vi "Action Point_Init.vi"(8 "error in":errorcluster, 11 "Action Point in":refnum<class "Action Point.lvclass">) -> (0 "error out":errorcluster, 3 "Action Point out":refnum<class "Action Point.lvclass">)   [LabVIEW 2024, in "Action Point.lvclass"]
uses:
  Action Point.lvclass
  Config from JSON/Config from JSON.lvclass
  D:/git/HAL/Source/Interfaces/IConfiguration/IConfiguration.lvclass
  Interfaces/IInitialize/IInitialize.lvclass
  Interfaces/ILog Data/ILog Data.lvclass
  Action Point.lvclass/Action Point.ctl
  Interfaces/IConfiguration/IConfiguration.lvclass
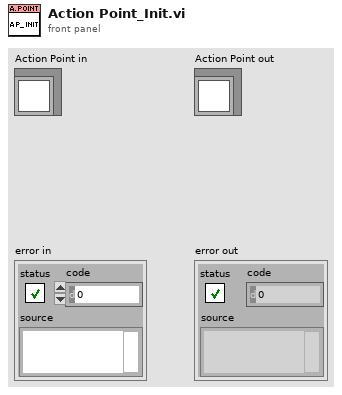
[diagram p1: front panel]
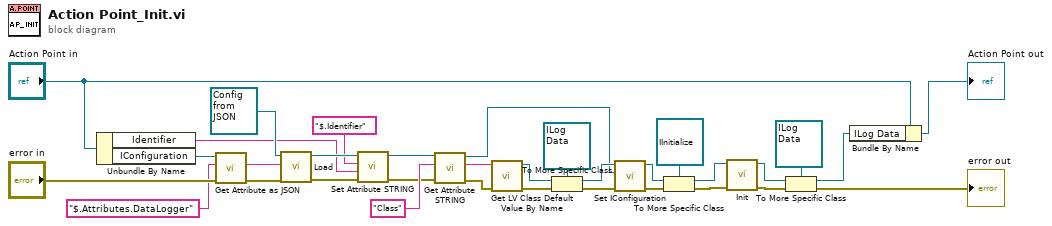
[diagram p0: block diagram]
diagram:
  n1 = Unbundle By Name("Action Point in") -> ("Identifier"=w1:string, "IConfiguration"=w22:refnum<class "IConfiguration.lvclass">)
  n2 = call-dynamic "Get Attribute as JSON.vi"("error in"="error in", "Attribute"="$.Attributes.DataLogger", "IConfiguration in"=w22) -> ("error out"=w20:errorcluster, "<JSON>"=w18:string)  [unwired: 6 in, 1 out]
  n3 = call-dynamic "Load.vi"("error in"=w20, "Source"=w18, "Config From JSON in"=refnum<class "Config from JSON.lvclass"> refnum) -> ("error out"=w16:errorcluster, "Config From JSON out"=w4:refnum<class "Config from JSON.lvclass">)  [unwired: 7 in]
  n4 = call-dynamic "Set Attribute STRING.vi"("error in"=w16, "Value"=w1, "Path"="$.Identifier", "Config from JSON in"=w4) -> ("error out"=w5:errorcluster, "Config from JSON out"=w3:refnum<class "Config from JSON.lvclass">)  [unwired: 6 in]
  n5 = call-dynamic "Get Attribute STRING.vi"("error in"=w5, "Attribute"="Class", "ConfigFromJSON in"=w3) -> ("error out"=w31:errorcluster, "Value"=w32:string, "ConfigFromJSON out"=w15:refnum<class "Config from JSON.lvclass">)  [unwired: 6 in]
  n6 = call <vilib>:"Get LV Class Default Value By Name.vi"("error in (no error)"=w31, "class name"=w32) -> ("error out"=w30:errorcluster, "object"=w28:refnum<class>)  [unwired: 8 in]
  n7 = To More Specific Class(target class=refnum<class "ILog Data.lvclass"> refnum ("ILog Data.lvclass"), reference=w28, error in=w30) -> (specific class reference=w23:refnum<class "ILog Data.lvclass">, error out=w25:errorcluster)
  n8 = call-dynamic "Set IConfiguration.vi"("error in"=w25, "IConfiguration"=w15, "IHasConfiguration in"=w23) -> ("error out"=w24:errorcluster, "IHasConfiguration out"=w13:refnum<class "ILog Data.lvclass">)  [unwired: 7 in]
  n9 = To More Specific Class(target class=refnum<class "IInitialize.lvclass"> refnum ("IInitialize.lvclass"), reference=w13, error in=w24) -> (specific class reference=w10:refnum<class "IInitialize.lvclass">, error out=w14:errorcluster)
  n10 = call-dynamic "Init.vi"("error in"=w14, "IInitialize in"=w10) -> ("error out"=w11:errorcluster, "IInitialize out"=w8:refnum<class "IInitialize.lvclass">)  [unwired: 8 in]
  n11 = To More Specific Class(target class=refnum<class "ILog Data.lvclass"> refnum ("ILog Data.lvclass"), reference=w8, error in=w11) -> (specific class reference=w6:refnum<class "ILog Data.lvclass">, error out=→"error out":errorcluster)
  n12 = Bundle By Name(cluster="Action Point in", "ILog Data"=w6) -> (→"Action Point out":refnum<class "Action Point.lvclass">)
